vi "AdditonalInputRead.vi"() -> ()   [LabVIEW 2019]
panel:
  out "1st Stage":dbl
  out "read buffer":string
  out "Waveform Chart":dbl[][](graph)
  out "D4":dbl
  out "D3":dbl
  out "Heater?":dbl
  out "Pot?":dbl
  out "Magnet?":dbl
  out "C3":dbl
  out "2nd Stage":dbl
  in  "VISA resource name":refnum<visa-resource-name>
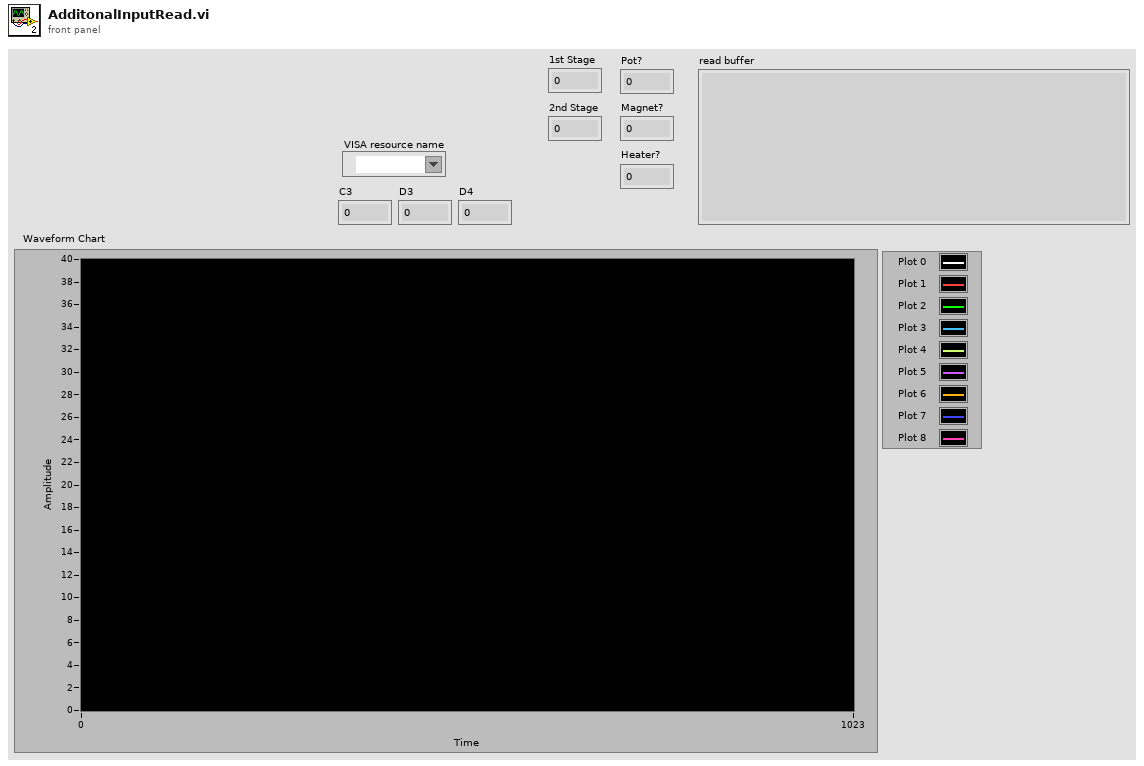
[diagram p1: front panel]
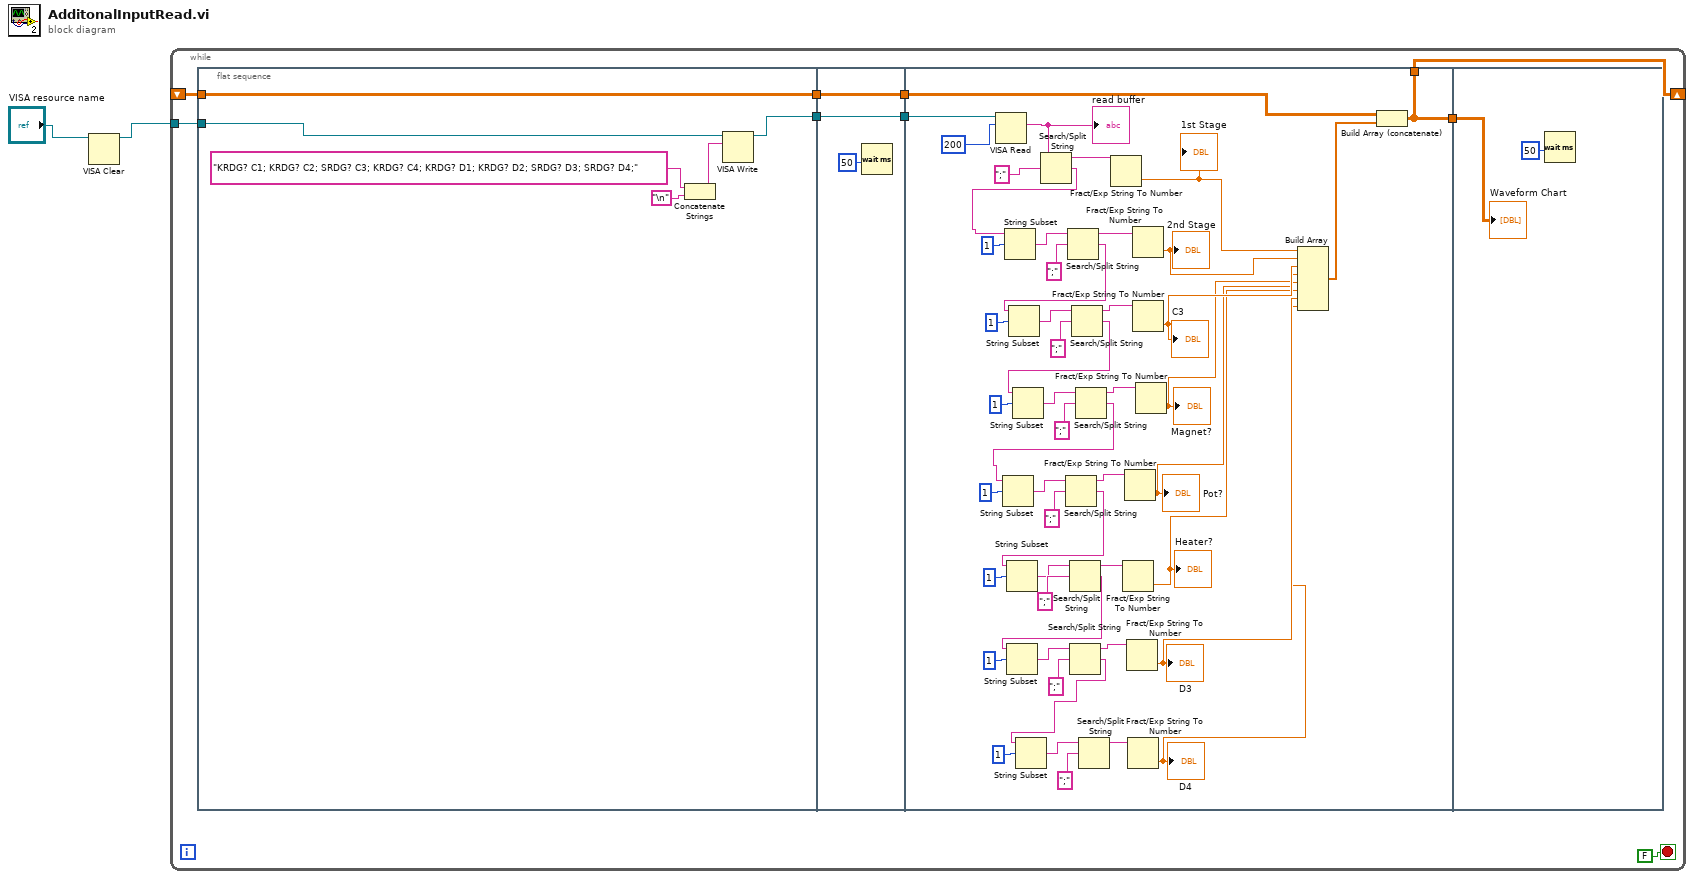
[diagram p0: block diagram]
diagram:
  n1 = VISA Clear(VISA resource name="VISA resource name") -> (VISA resource name out=w2:refnum<visa-resource-name>)  [unwired: 1 in, 1 out]
  n2 = while {
    tunnel: w2 -> [w9]
    shift-right: [w5] -> _
    shift-left: _ -> [w8]
    stop <- FALSE stop-if-true
    n3 = flat-sequence {
      tunnel: [w17] -> w11
      tunnel: w9 -> [w16]
      tunnel: w8 -> [w12]
      tunnel: [w12] -> w6
      tunnel: w11 -> [w20]
      tunnel: [w20] -> w10
      tunnel: [w18] -> w7
      tunnel: w6 -> [w18]
      tunnel: w10 -> [w70]
      tunnel: w7 -> [w24]
      tunnel: [w22] -> w5
      tunnel: [w22] -> w4
      tunnel: w4 -> [w72]
      frame #0 {
        n4 = Concatenate Strings("KRDG? C1; KRDG? C2; SRDG? C3; KRDG? C4; KRDG? D1; KRDG? D2; SRDG? D3; SRDG? D4;", "\n") -> (w13:string)
        n5 = VISA Write(VISA resource name=w16, write buffer=w13) -> (VISA resource name out=w17:refnum<visa-resource-name>)  [unwired: 1 in, 2 out]
      }
      frame #1 {
        n6 = Wait (ms)(milliseconds to wait=50) -> ()  [unwired: 1 out]
      }
      frame #2 {
        n7 = VISA Read(VISA resource name=w70, byte count=200) -> (read buffer=w69:string)  [unwired: 1 in, 3 out]
        "read buffer" <- w69
        n8 = Search/Split String(string=w69, search string/char (-)=";") -> (substring before match=w39:string, match + rest of string=w66:string)  [unwired: 1 in, 1 out]
        n9 = String Subset(string=w66, offset (0)=u32 1 ("byte count")) -> (substring=w64:string)  [unwired: 1 in]
        n10 = Search/Split String(string=w64, search string/char (-)=";") -> (substring before match=w38:string, match + rest of string=w45:string)  [unwired: 1 in, 1 out]
        n11 = String Subset(string=w45, offset (0)=u32 1 ("byte count")) -> (substring=w61:string)  [unwired: 1 in]
        n12 = Search/Split String(string=w61, search string/char (-)=";") -> (substring before match=w37:string, match + rest of string=w44:string)  [unwired: 1 in, 1 out]
        n13 = String Subset(string=w44, offset (0)=u32 1 ("byte count")) -> (substring=w58:string)  [unwired: 1 in]
        n14 = Search/Split String(string=w58, search string/char (-)=";") -> (substring before match=w36:string, match + rest of string=w43:string)  [unwired: 1 in, 1 out]
        n15 = String Subset(string=w43, offset (0)=u32 1 ("byte count")) -> (substring=w55:string)  [unwired: 1 in]
        n16 = Search/Split String(string=w55, search string/char (-)=";") -> (substring before match=w35:string, match + rest of string=w42:string)  [unwired: 1 in, 1 out]
        n17 = String Subset(string=w42, offset (0)=u32 1 ("byte count")) -> (substring=w52:string)  [unwired: 1 in]
        n18 = Search/Split String(string=w52, search string/char (-)=";") -> (substring before match=w34:string, match + rest of string=w41:string)  [unwired: 1 in, 1 out]
        n19 = String Subset(string=w41, offset (0)=u32 1 ("byte count")) -> (substring=w49:string)  [unwired: 1 in]
        n20 = Search/Split String(string=w49, search string/char (-)=";") -> (substring before match=w33:string, match + rest of string=w40:string)  [unwired: 1 in, 1 out]
        n21 = String Subset(string=w40, offset (0)=u32 1 ("byte count")) -> (substring=w46:string)  [unwired: 1 in]
        n22 = Search/Split String(string=w46, search string/char (-)=";") -> (substring before match=w32:string)  [unwired: 1 in, 2 out]
        n23 = Fract/Exp String To Number(string=w39) -> (number=w31:dbl)  [unwired: 3 in, 1 out]
        "1st Stage" <- w31
        n24 = Fract/Exp String To Number(string=w34) -> (number=w21:dbl)  [unwired: 3 in, 1 out]
        "Heater?" <- w21
        n25 = Fract/Exp String To Number(string=w35) -> (number=w27:dbl)  [unwired: 3 in, 1 out]
        "Pot?" <- w27
        n26 = Fract/Exp String To Number(string=w33) -> (number=w26:dbl)  [unwired: 3 in, 1 out]
        "D3" <- w26
        n27 = Fract/Exp String To Number(string=w32) -> (number=w25:dbl)  [unwired: 3 in, 1 out]
        "D4" <- w25
        n28 = Fract/Exp String To Number(string=w38) -> (number=w30:dbl)  [unwired: 3 in, 1 out]
        "2nd Stage" <- w30
        n29 = Fract/Exp String To Number(string=w37) -> (number=w29:dbl)  [unwired: 3 in, 1 out]
        "C3" <- w29
        n30 = Fract/Exp String To Number(string=w36) -> (number=w28:dbl)  [unwired: 3 in, 1 out]
        "Magnet?" <- w28
        n31 = Build Array(w31, w30, w29, w28, w27, w21, w26, w25) -> (w23:dbl[])
        n32 = Build Array (concatenate)(w24, w23) -> (w22:dbl[][])
      }
      frame #3 {
        n33 = Wait (ms)(milliseconds to wait=50) -> ()  [unwired: 1 out]
        "Waveform Chart" <- w72
      }
    }
  }
